vi "GetAnalyzerVisibleName.vi"(8 "error in":errorcluster, 11 "connection ID in":refnum<k5>) -> (0 "error out":errorcluster, 1 "Error Info":T1, 2 "Analyzer Visible Name":string, 3 "connection ID out":refnum<k5>, 4 "Log String":string, 5 "OK":bool)   [LabVIEW 2020, in "ProdigyRemoteControl.lvlib"]
uses:
  ProdigyRemoteControl.lvlib
  DEFINITIONS/DEF_RcError.ctl
  DEFINITIONS/DEF_RcCmd.ctl
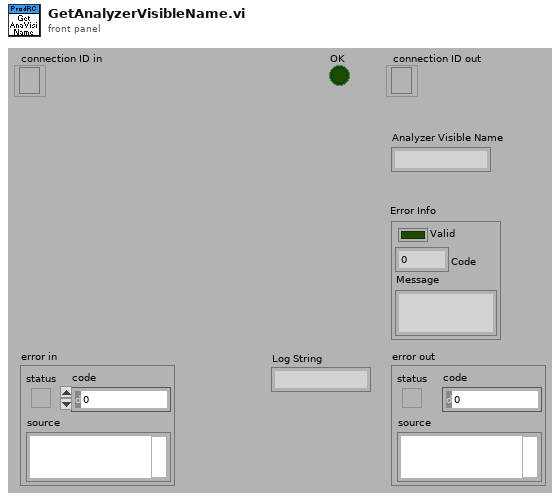
[diagram p1: front panel]
types:
  T1 = typedef "ProdigyRemoteControl.lvlib/DEF_RcError.ctl" = cluster{"Valid":bool, "Code":u16, "Message":string}
  T2 = typedef "ProdigyRemoteControl.lvlib/DEF_RcCmd.ctl" = string
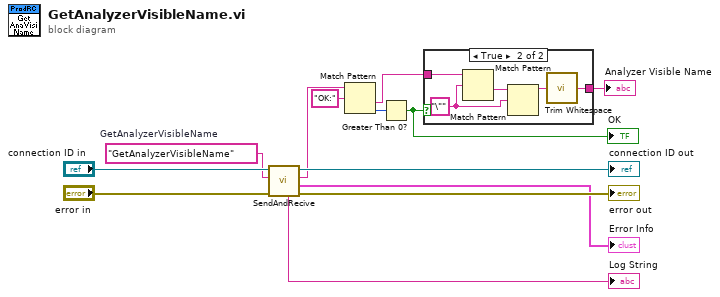
[diagram p0: block diagram]
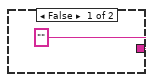
[diagram p2: hidden frame]
diagram:
  w9 = T2 "GetAnalyzerVisibleName"  # GetAnalyzerVisibleName
  n1 = call "SendAndRecive.vi"("error in"="error in", "Command"=w9, "connection ID in"="connection ID in") -> ("error out"=→"error out":errorcluster, "Error Info"=→"Error Info":T1, "Answer"=w5:string, "connection ID out"=→"connection ID out":refnum<k5>, "Log String"=→"Log String":string)  [unwired: 4 in]
  n2 = Match Pattern(string=w5, regular expression="OK:") -> (after substring=w3:string, offset past match=w4:i32)  [unwired: 1 in, 2 out]
  n3 = Greater Than 0?(x=w4) -> (x > 0?=w2:bool)
  "OK" <- w2
  n4 = case shown="True" w2 {
    tunnel: ["" ("Value") w15] -> w1
    tunnel: w3 -> [_ w16]
    frame False {
    }
    frame True {
      w18 = "\"" ("regular expression")
      n5 = Match Pattern(string=w16, regular expression=w18) -> (after substring=w19:string)  [unwired: 1 in, 3 out]
      n6 = Match Pattern(string=w19, regular expression=w18) -> (before substring=w17:string)  [unwired: 1 in, 3 out]
      n7 = call <vilib>:"Trim Whitespace.vi"("string"=w17) -> ("trimmed string"=w15:string)  [unwired: 1 in]
    }
  }
  "Analyzer Visible Name" <- w1
